vi "n4tobob1.vi"() -> ()   [LabVIEW 2014, in "Panels.lvlib"]
uses:
  Panels.lvlib
  CSlibraries-extern/DimLVEvent/DimIndicators/DimIndicators.lvlib
  CS_Core/CSSystem/CoreLib/CoreLib.lvlib
  CSlibraries/UtilityLib/UtilityLib.valueStatus.ctl
  CSlibraries/UtilityLib/UtilityLib.lvlib
  CSlibraries-extern/DimLVEvent/LVDimInterface/LVDimInterface.lvlib
  Instance           1 16Saved   n4tobob1 .vi
  CSlibraries-extern/DimLVEvent/DimIndicators/DimIndicators.numericType.ctl
  CSlibraries-extern/DimLVEvent/DimIndicators/DimIndicators.numericArrayType.ctl
  CSlibraries-extern/DimLVEvent/DimIndicators/DimIndicators.anyType.ctl
panel:
  in  "SetFileLocation_Data":T1={"data"="NOLINK", "no link"=TRUE, "quality"=-1, "timeStamp"=0.0}
  in  "LN4Accel2":bool
  in  "LN4Accel3":bool
  in  "LN4DefY":bool
  in  "LN4DefX":bool
  in  "10DegDefX":bool
  in  "ELens0":bool
  out "LN4Accel3_Mon":dbl=inf format="%.4f"
  out "LN4Accel2_Mon":dbl=inf format="%.4f"
  out "i ref out":refnum<vi>
  in  "Last Loaded File_Data":T1
  out "FileUpToDate":bool caption="Parameter Changed"
  in  "Close All Panels":bool
  in  "LN4Accel2_SetValueInfoData":T2
  in  "LN4Accel3_SetValueInfoData":T2
  in  "ELens0_SetValueInfoData":T2
  in  "LN4DefX_SetValueInfoData":T2
  in  "LN4DefY_SetValueInfoData":T2
  in  "10DegDefX_SetValueInfoData":T2
  in  "10DegDefX_SetData":T2
  in  "LN4DefY_SetData":T2
  in  "LN4DefX_SetData":T2
  in  "ELens0_SetData":T2
  in  "LN4Accel3_SetData":T2
  in  "LN4Accel2_SetData":T2
  out "Last Loaded File":string
  in  "SetFileLocation":path=path "\\\\intranet\\Files/projects/lebit/Data Exchange/data/N4tobob1Control"
  in  "10DegDefY_MonData":T3={"data"=inf, "no link"=FALSE, "quality"=1, "timeStamp"=3262371343.476}
  in  "10DegDefX_MonData":T3={"data"=inf, "no link"=FALSE, "quality"=1, "timeStamp"=3262371343.476}
  in  "LN4DefY_MonData":T3={"data"=inf, "no link"=FALSE, "quality"=1, "timeStamp"=3262371343.476}
  in  "LN4DefX_MonData":T3={"data"=inf, "no link"=FALSE, "quality"=1, "timeStamp"=3262371343.476}
  in  "ELens0_MonData":T3={"data"=inf, "no link"=FALSE, "quality"=1, "timeStamp"=3262371343.46}
  in  "LN4Accel3_MonData":T3={"data"=inf, "no link"=FALSE, "quality"=1, "timeStamp"=3262371343.46}
  in  "LN4Accel2_MonData":T3={"data"=inf, "no link"=FALSE, "quality"=1, "timeStamp"=3262371343.46}
  out "LN4DefX_Mon":dbl=inf format="%.4f"
  out "10DegDefY_Mon":dbl=inf format="%.4f"
  out "10DegDefX_Mon":dbl=inf format="%.4f"
  out "LN4DefY_Mon":dbl=inf format="%.4f"
  out "ELens0_Mon":dbl=inf format="%.4f"
  # "Parameter changed, data file is no longer up-to-date."
  # "10DegDefY"
  # "LN4Accel1 = DC8"
  # "LN4Accel4 =-5kV"
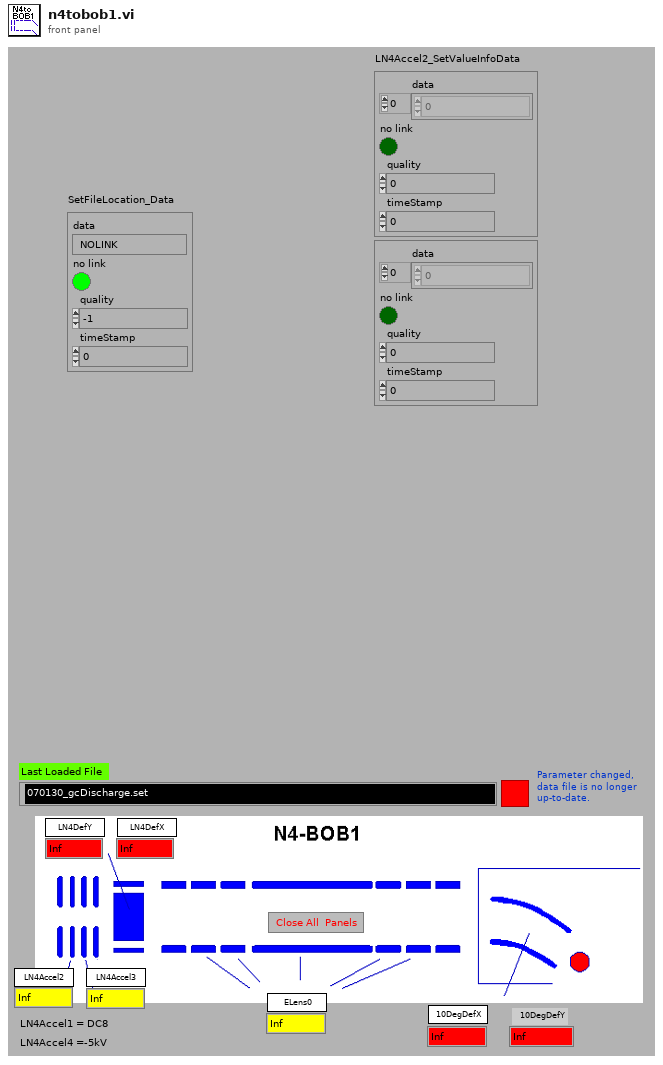
[diagram p1: front panel]
types:
  T1 = typedef "DimIndicators.lvlib/DimIndicators.anyType.ctl" = cluster{"data":string, "no link":bool, "quality":i32, "timeStamp":dbl}
  T2 = typedef "DimIndicators.lvlib/DimIndicators.numericArrayType.ctl" = cluster{"data":dbl[], "no link":bool, "quality":i32, "timeStamp":dbl}
  T3 = typedef "DimIndicators.lvlib/DimIndicators.numericType.ctl" = cluster{"data":dbl, "no link":bool, "quality":i32, "timeStamp":dbl}
  T4 = typedef "UtilityLib.lvlib/UtilityLib.valueStatus.ctl" = enum16{"no info available", "stand by/off", "on", "warning", "alarm/malfunction", "not implemented", "user action required", "important information", "system default", "control default", "indicator default", "button default"}
  T5 = cluster{"data":string, "no link":bool, "quality":i32, "timeStamp":dbl}
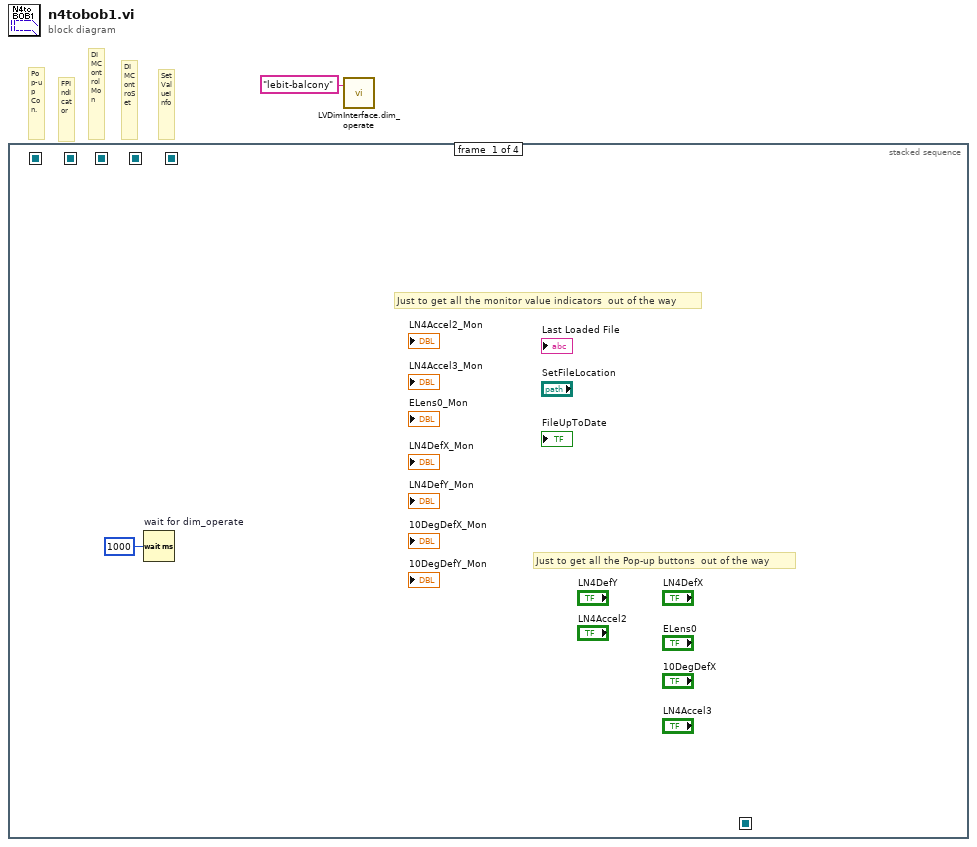
[diagram p0: block diagram]
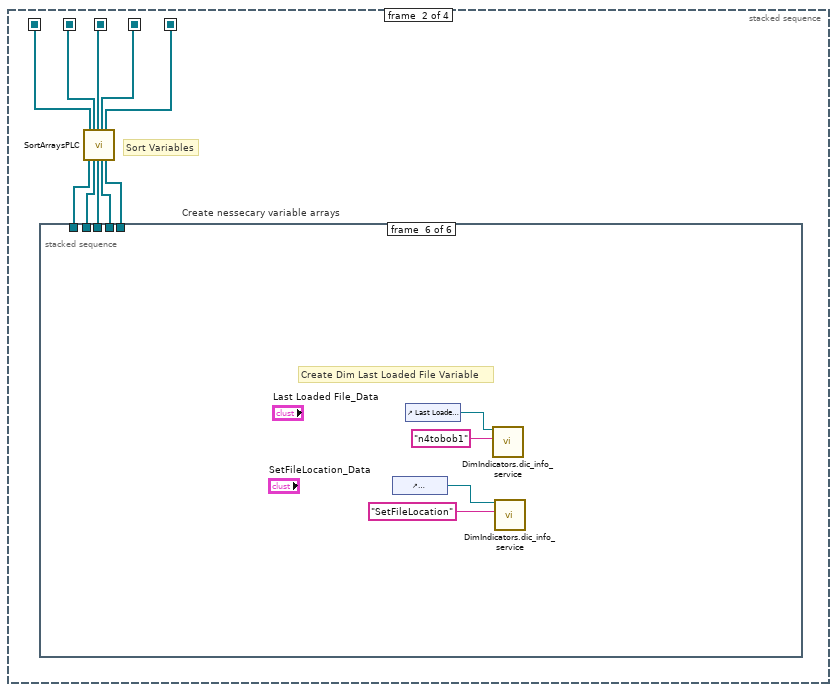
[diagram p2: hidden frame]
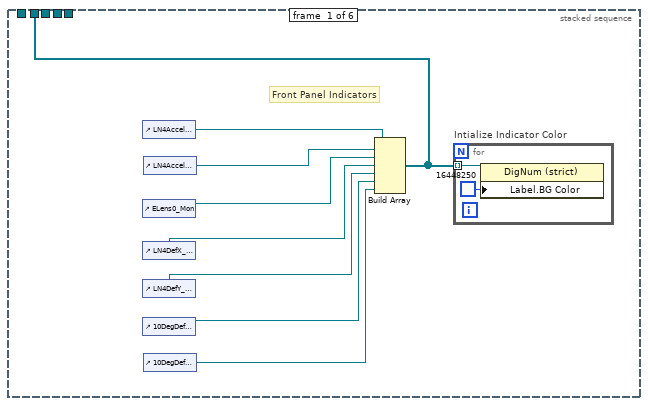
[diagram p3: hidden frame]
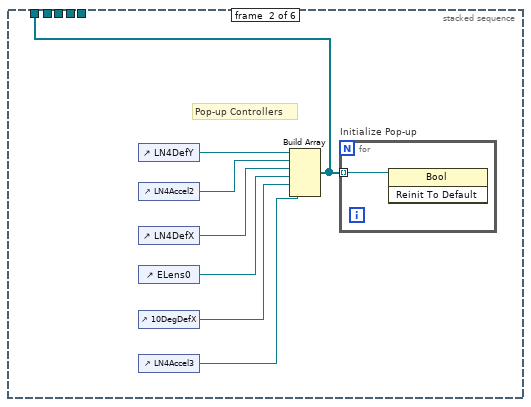
[diagram p4: hidden frame]
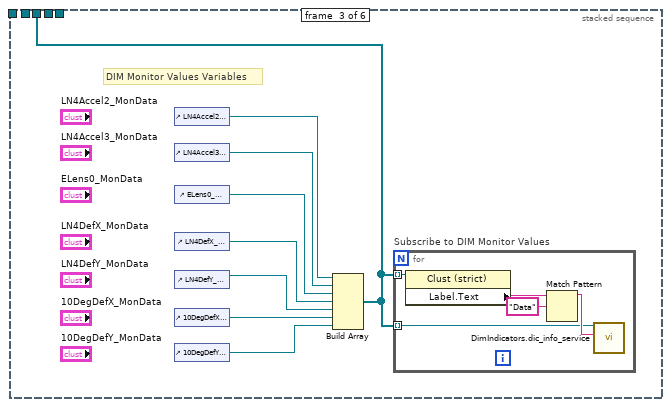
[diagram p5: hidden frame]
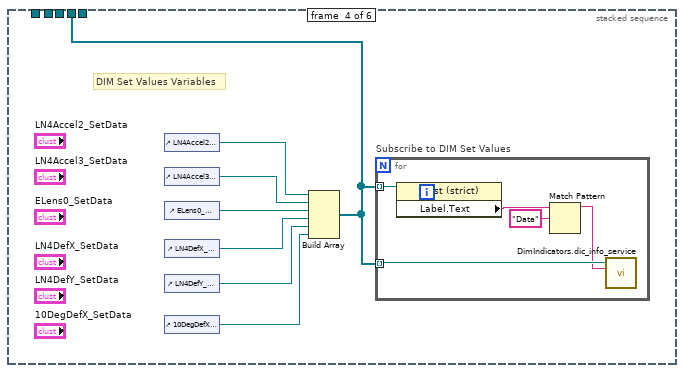
[diagram p6: hidden frame]
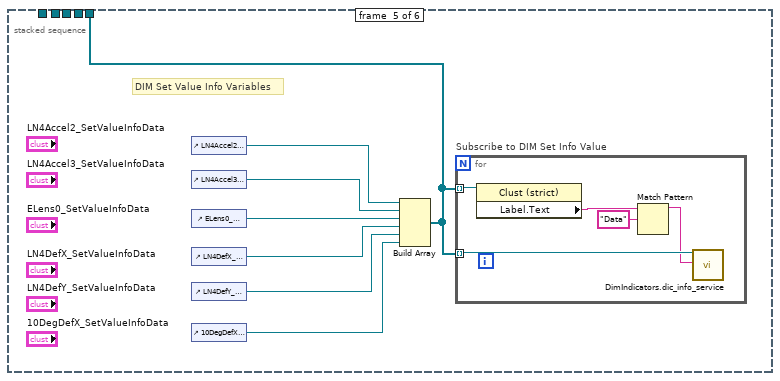
[diagram p7: hidden frame]
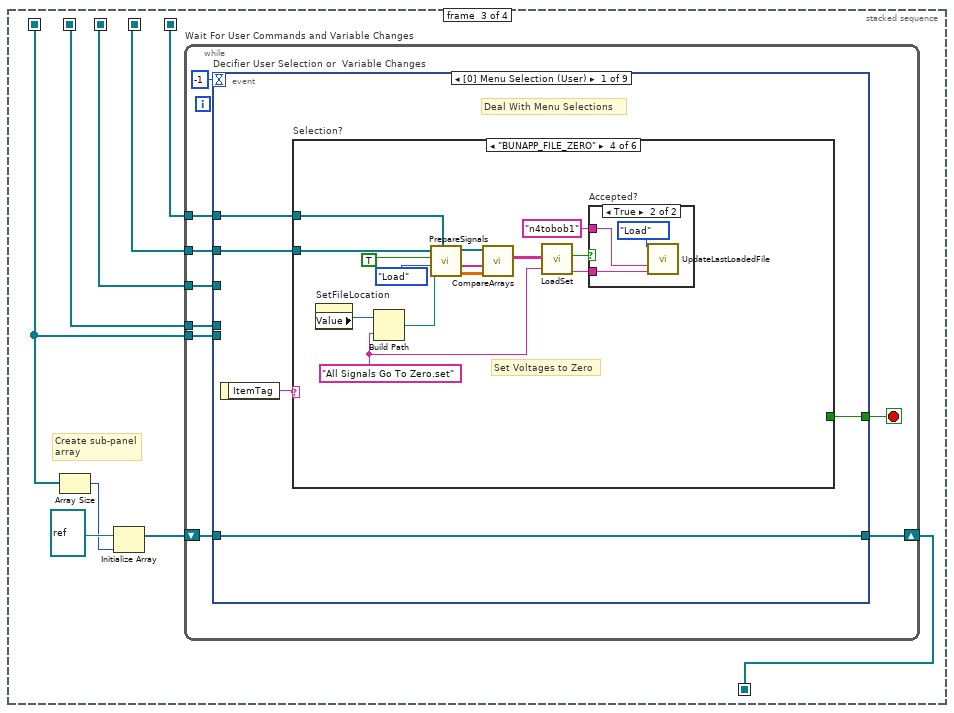
[diagram p8: hidden frame]
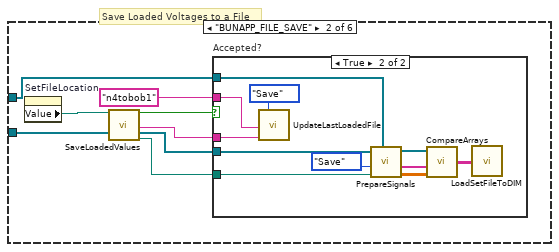
[diagram p10: hidden frame]
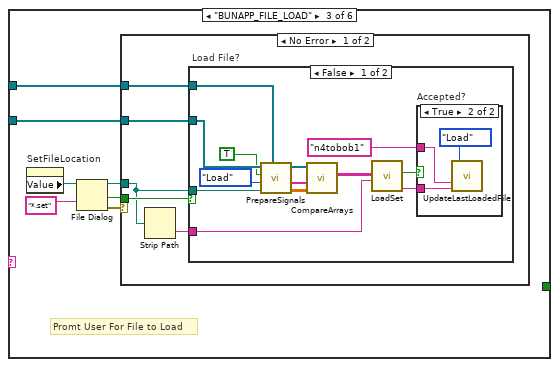
[diagram p12: hidden frame]
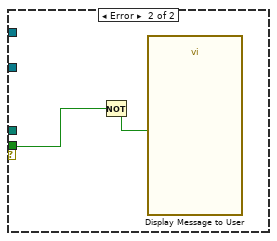
[diagram p15: hidden frame]
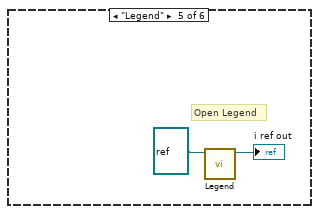
[diagram p17: hidden frame]
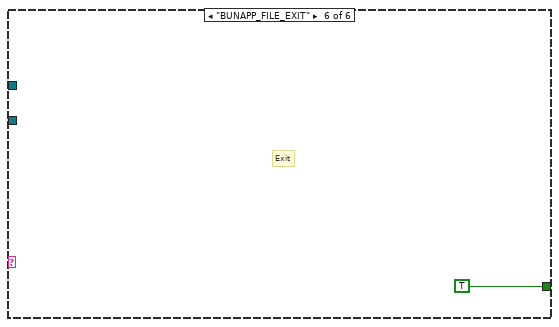
[diagram p18: hidden frame]
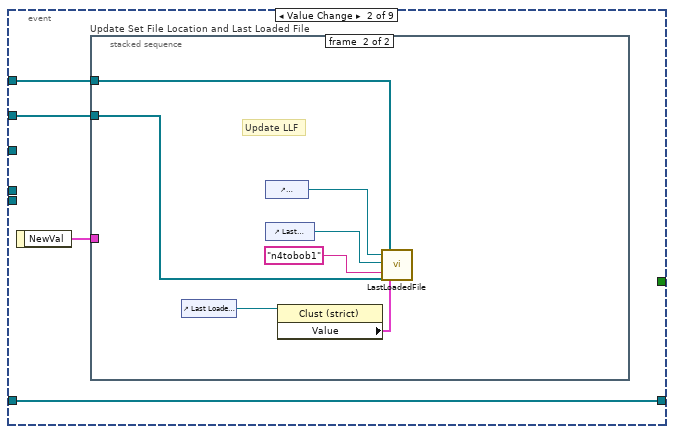
[diagram p19: hidden frame]
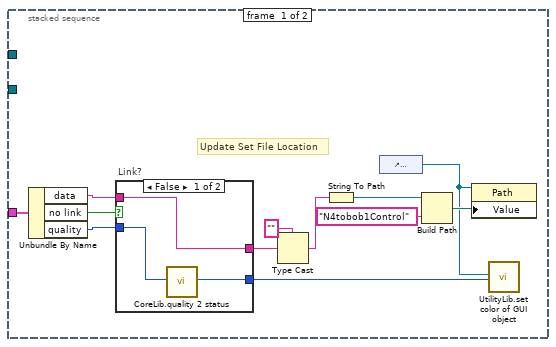
[diagram p20: hidden frame]
diagram:
  # "Pop-up Con."
  # "SetValueInfo"
  # "DIMControSet"
  # "DIMControlMon"
  # "FPIndicator"
  n1 = stacked-sequence {
    seq-local: [_ w11 _ _] -> [_ _ w77 _]
    seq-local: [_ w10 _ _] -> [_ _ w80 w273]
    seq-local: [_ _ w75 _] -> [_ _ _ w272]
    seq-local: [_ w9 _ _] -> [_ _ w74 w271]
    seq-local: [_ w8 _ _] -> [_ _ w73 w270]
    seq-local: [_ w12 _ _] -> [_ _ w72 _]
    frame #0 {
      # "Just to get all the Pop-up buttons  out of the way"
      # "Just to get all the monitor value indicators  out of the way"
      n2 = Wait (ms) "wait for dim_operate"(milliseconds to wait=u32 1000) -> ()  [unwired: 1 out]
    }
    frame #1 {
      # "Sort Variables"
      n3 = stacked-sequence "Create nessecary variable arrays" {
        tunnel: [w13 _ _ _ _ _] -> w7
        tunnel: [_ w23 _ _ _ _] -> w6
        tunnel: [_ _ w31 _ _ _] -> w5
        tunnel: [_ _ _ w44 _ _] -> w4
        tunnel: [_ _ _ _ w56 _] -> w3
        frame #0 {
          # "Front Panel Indicators"
          n4 = control-ref of="LN4Accel2_Mon"() -> (w15:refnum<vi>)
          n5 = control-ref of="ELens0_Mon"() -> (w20:refnum<vi>)
          n6 = control-ref of="LN4DefX_Mon"() -> (w19:refnum<vi>)
          n7 = control-ref of="LN4DefY_Mon"() -> (w18:refnum<vi>)
          n8 = control-ref of="10DegDefX_Mon"() -> (w17:refnum<vi>)
          n9 = control-ref of="LN4Accel3_Mon"() -> (w14:refnum<vi>)
          n10 = control-ref of="10DegDefY_Mon"() -> (w16:refnum<vi>)
          n11 = Build Array(w15, w14, w20, w19, w18, w17, w16) -> (w13:refnum<vi>[])
          n12 = for "Intialize Indicator Color" {
            tunnel: w13 -> [w22] mode=indexing
            n13 = property class="DigNum (strict)"(reference=w22, "Label.BG Color"=u32 16448250 ("Color Box")) -> ()  [unwired: 1 in, 2 out]
          }
        }
        frame #1 {
          # "Pop-up Controllers"
          n14 = control-ref of="LN4DefY"() -> (w29:refnum<vi>)
          n15 = control-ref of="LN4Accel2"() -> (w28:refnum<vi>)
          n16 = control-ref of="LN4DefX"() -> (w27:refnum<vi>)
          n17 = control-ref of="ELens0"() -> (w26:refnum<vi>)
          n18 = control-ref of="10DegDefX"() -> (w25:refnum<vi>)
          n19 = control-ref of="LN4Accel3"() -> (w24:refnum<vi>)
          n20 = Build Array(w29, w28, w27, w26, w25, w24) -> (w23:refnum<vi>[])
          n21 = for "Initialize Pop-up" {
            tunnel: w23 -> [w30] mode=indexing
            n22 = invoke class="Bool" method="Reinit To Default"(reference=w30) -> ()  [unwired: 2 in, 3 out]
          }
        }
        frame #2 {
          # "DIM Monitor Values Variables"
          n23 = control-ref of="LN4Accel2_MonData"() -> (w38:refnum<vi>)
          n24 = control-ref of="LN4Accel3_MonData"() -> (w37:refnum<vi>)
          n25 = control-ref of="ELens0_MonData"() -> (w36:refnum<vi>)
          n26 = control-ref of="LN4DefX_MonData"() -> (w35:refnum<vi>)
          n27 = control-ref of="LN4DefY_MonData"() -> (w34:refnum<vi>)
          n28 = control-ref of="10DegDefX_MonData"() -> (w33:refnum<vi>)
          n29 = control-ref of="10DegDefY_MonData"() -> (w32:refnum<vi>)
          n30 = Build Array(w38, w37, w36, w35, w34, w33, w32) -> (w31:refnum<vi>[])
          n31 = for "Subscribe to DIM Monitor Values" {
            tunnel: w31 -> [w40] mode=indexing
            tunnel: w31 -> [w39] mode=indexing
            n32 = property class="Clust (strict)"(reference=w39) -> ("Label.Text"=w42:string)  [unwired: 1 in, 2 out]
            n33 = Match Pattern(string=w42, regular expression="Data") -> (before substring=w41:string)  [unwired: 1 in, 3 out]
            n34 = call "DimIndicators.dic_info_service.vi"("controlRef"=w40, "serviceName"=w41) -> ()  [unwired: 16 in, 2 out]
          }
        }
        frame #3 {
          # "DIM Set Values Variables"
          n35 = control-ref of="LN4Accel2_SetData"() -> (w50:refnum<vi>)
          n36 = control-ref of="LN4Accel3_SetData"() -> (w49:refnum<vi>)
          n37 = control-ref of="ELens0_SetData"() -> (w48:refnum<vi>)
          n38 = control-ref of="LN4DefX_SetData"() -> (w47:refnum<vi>)
          n39 = control-ref of="LN4DefY_SetData"() -> (w46:refnum<vi>)
          n40 = control-ref of="10DegDefX_SetData"() -> (w45:refnum<vi>)
          n41 = Build Array(w50, w49, w48, w47, w46, w45) -> (w44:refnum<vi>[])
          n42 = for "Subscribe to DIM Set Values" {
            tunnel: w44 -> [w51] mode=indexing
            tunnel: w44 -> [w55] mode=indexing
            n43 = property class="Clust (strict)"(reference=w51) -> ("Label.Text"=w54:string)  [unwired: 1 in, 2 out]
            n44 = Match Pattern(string=w54, regular expression="Data") -> (before substring=w52:string)  [unwired: 1 in, 3 out]
            n45 = call "DimIndicators.dic_info_service.vi"("controlRef"=w55, "serviceName"=w52) -> ()  [unwired: 16 in, 2 out]
          }
        }
        frame #4 {
          # "DIM Set Value Info Variables"
          n46 = control-ref of="LN4Accel2_SetValueInfoData"() -> (w62:refnum<vi>)
          n47 = control-ref of="LN4Accel3_SetValueInfoData"() -> (w61:refnum<vi>)
          n48 = control-ref of="ELens0_SetValueInfoData"() -> (w60:refnum<vi>)
          n49 = control-ref of="LN4DefX_SetValueInfoData"() -> (w59:refnum<vi>)
          n50 = control-ref of="LN4DefY_SetValueInfoData"() -> (w58:refnum<vi>)
          n51 = control-ref of="10DegDefX_SetValueInfoData"() -> (w57:refnum<vi>)
          n52 = Build Array(w62, w61, w60, w59, w58, w57) -> (w56:refnum<vi>[])
          n53 = for "Subscribe to DIM Set Info Value" {
            tunnel: w56 -> [w63] mode=indexing
            tunnel: w56 -> [w67] mode=indexing
            n54 = property class="Clust (strict)"(reference=w63) -> ("Label.Text"=w66:string)  [unwired: 1 in, 2 out]
            n55 = Match Pattern(string=w66, regular expression="Data") -> (before substring=w64:string)  [unwired: 1 in, 3 out]
            n56 = call "DimIndicators.dic_info_service.vi"("controlRef"=w67, "serviceName"=w64) -> ()  [unwired: 16 in, 2 out]
          }
        }
        frame #5 {
          # "Create Dim Last Loaded File Variable"
          n57 = control-ref of="SetFileLocation_Data"() -> (w71:refnum<vi>)
          n58 = control-ref of="Last Loaded File_Data"() -> (w69:refnum<vi>)
          n59 = call "DimIndicators.dic_info_service.vi"("controlRef"=w69, "serviceName"="n4tobob1" ("string")) -> ()  [unwired: 16 in, 2 out]
          n60 = call "DimIndicators.dic_info_service.vi"("controlRef"=w71, "serviceName"="SetFileLocation" ("string")) -> ()  [unwired: 16 in, 2 out]
        }
      }
      n61 = call "SortArraysPLC.vi"("Pop-up Con."=w6, "FPIndicator in"=w7, "DIMControlMon"=w5, "DIMControSet"=w4, "SetValueInfo"=w3) -> ("Pop-up Con. out"=w12:refnum<vi>[], "FPIndicator out"=w11:refnum<vi>[], "DIMControlMon out"=w10:refnum<vi>[], "DIMControSet out"=w9:refnum<vi>[], "SetValueInfo out"=w8:refnum<vi>[])  [unwired: 18 in]
    }
    frame #2 {
      # "Create sub-panel\narray"
      n62 = Array Size(array=w72) -> (size(s)=w76:i32)
      n63 = Initialize Array(refnum<vi> refnum ("vi reference"), w76) -> (w79:refnum<vi>[])
      n64 = while "Wait For User Commands and Variable Changes" {
        tunnel: w80 -> [w88]
        tunnel: w77 -> [w87]
        shift-right: [w85] -> w75
        shift-left: w79 -> [w86]
        tunnel: w74 -> [w84]
        tunnel: w73 -> [w83]
        tunnel: w72 -> [w81]
        stop <- w89 stop-if-true
        n65 = event "Decifier User Selection or  Variable Changes" shown="[0] Menu Selection (User)" {
          selector: _ -> [_ _ _ _ _ _ _ _ _]
          dyn-events: _ -> [_ _ _ _ _ _ _ _ _]
          timeout: -1 -> [_ _ _ _ _ _ _ _ _]
          tunnel: [w91 _ _ _ _ _ _ _ TRUE ("stop")] -> w89
          tunnel: w88 -> [_ _ _ w203 _ _ _ _ w246]
          tunnel: w87 -> [_ _ _ w202 _ _ _ _ _]
          tunnel: w86 -> [w94 w165 w198 w205 w223 w231 w238 w244 w245]
          tunnel: [w94 w165 w198 w205 w223 w229 w236 w244 _] -> w85
          tunnel: w84 -> [w92 w166 w195 _ w221 _ _ _ w247]
          tunnel: w83 -> [w90 w164 w192 _ _ _ _ _ w248]
          tunnel: w81 -> [_ _ _ _ _ w225 _ _ _]
          event Menu Selection (User) {
            # "Deal With Menu Selections"
            n66 = event-data() -> ("ItemTag"=w93:string)  [unwired: 1 in]
            n67 = case "Selection?" shown="\"BUNAPP_FILE_ZERO\"" w93 {
              tunnel: w92 -> [_ w99 w119 w157 _ _]
              tunnel: [_ _ _ _ _ TRUE ("stop")] -> w91
              tunnel: w90 -> [_ w95 w114 w144 _ _]
              frame "False", Default {
              }
              frame "BUNAPP_FILE_SAVE" {
                # "Save Loaded Voltages to a File"
                n68 = property on="SetFileLocation" class="Path"() -> ("Value"=w100:path)  [unwired: 2 in, 2 out]
                n69 = call "SaveLoadedValues.vi"("Panel Location?"=w100, "DIMControlSet in"=w99) -> ("File Saved?"=w101:bool, "File Name"=w98:string, "DIMControlSet out"=w96:refnum<vi>[], "Path"=w97:path)  [unwired: 14 in]
                n70 = case "Accepted?" shown="True" w101 {
                  tunnel: w98 -> [_ w111]
                  tunnel: "n4tobob1" ("string") -> [_ w113]
                  tunnel: w96 -> [_ w112]
                  tunnel: w97 -> [_ w110]
                  tunnel: w95 -> [_ w104]
                  frame False {
                  }
                  frame True {
                    n71 = call "UpdateLastLoadedFile.vi"("LoadOrSave"=enum16{"Load", "Save"}."Save", "GUIName"=w113, "FileNameIn"=w111) -> ()  [unwired: 13 in]
                    n72 = call "PrepareSignals.vi"("SetValueInfo in"=w104, "setfile path"=w110, "Enum"=enum16{"Save", "Load"}."Save", "DIMControSet in"=w112) -> ("indexed loaded Array"=w108:dbl[][], "Name Array"=w109:string[], "DIMControSet out"=w107:refnum<vi>[])  [unwired: 5 in]
                    n73 = call "CompareArrays.vi"("indexed loaded Array"=w108, "Name Array"=w109, "DIMControSet"=w107) -> ("Table for loading values"=w106:string[][])  [unwired: 4 in]
                    n74 = call "LoadSetFileToDIM.vi"("output array"=w106) -> ()  [unwired: 2 in]
                  }
                }
              }
              frame "BUNAPP_FILE_LOAD" {
                # "Promt User For File to Load"
                n75 = property on="SetFileLocation" class="Path"() -> ("Value"=w116:path)  [unwired: 2 in, 2 out]
                n76 = File Dialog(6:"*.set" ("pattern (all files)"), 11:w116) -> (0:w115:errorcluster, 1:w120:bool, 3:w117:path)  [unwired: 5 in, 1 out]
                n77 = case shown="No Error" w115 {
                  tunnel: w120 -> [w125 w142]
                  tunnel: w119 -> [w124 _]
                  tunnel: w117 -> [w122 _]
                  tunnel: w114 -> [w121 _]
                  frame No Error {
                    n78 = Strip Path(path=w122) -> (name=w123:string)  [unwired: 1 out]
                    n79 = case "Load File?" shown="False" w125 {
                      tunnel: w124 -> [w138 _]
                      tunnel: w123 -> [w132 _]
                      tunnel: w122 -> [w133 _]
                      tunnel: w121 -> [w126 _]
                      frame False {
                        n80 = call "PrepareSignals.vi"("SetValueInfo in"=w126, "setfile path"=w133, "Enum"=enum16{"Save", "Load"}."Load", "Display Message to \nUser"=TRUE ("Display Message to \nUser"), "DIMControSet in"=w138) -> ("indexed loaded Array"=w136:dbl[][], "Name Array"=w135:string[], "DIMControSet out"=w137:refnum<vi>[])  [unwired: 4 in]
                        n81 = call "CompareArrays.vi"("indexed loaded Array"=w136, "Name Array"=w135, "DIMControSet"=w137) -> ("Table for loading values"=w134:string[][])  [unwired: 4 in]
                        n82 = call "LoadSet.vi"("File Name In"=w132, "output array"=w134) -> ("File Name out"=w131:string, "Accepted"=w130:bool)  [unwired: 8 in]
                        n83 = case "Accepted?" shown="True" w130 {
                          tunnel: w131 -> [_ w141]
                          tunnel: "n4tobob1" ("string") -> [_ w140]
                          frame False {
                          }
                          frame True {
                            n84 = call "UpdateLastLoadedFile.vi"("LoadOrSave"=enum16{"Load", "Save"}."Load", "GUIName"=w140, "FileNameIn"=w141) -> ()  [unwired: 13 in]
                          }
                        }
                      }
                      frame True {
                      }
                    }
                  }
                  frame Error {
                    n85 = Not(x=w142) -> (.not. x?=w143:bool)
                    n86 = call "Display Message to User"("Enable"=w143) -> ()  [unwired: 9 in, 2 out]
                  }
                }
              }
              frame "BUNAPP_FILE_ZERO" {
                w148 = "All Signals Go To Zero.set" ("File Name")
                # "Set Voltages to Zero"
                n87 = property on="SetFileLocation" class="Path"() -> ("Value"=w146:path)  [unwired: 2 in, 2 out]
                n88 = Build Path(base path=w146, name or relative path=w148) -> (appended path=w147:path)
                n89 = call "PrepareSignals.vi"("SetValueInfo in"=w144, "setfile path"=w147, "Enum"=enum16{"Save", "Load"}."Load", "Display Message to \nUser"=TRUE ("Display Message to \nUser"), "DIMControSet in"=w157) -> ("indexed loaded Array"=w155:dbl[][], "Name Array"=w154:string[], "DIMControSet out"=w156:refnum<vi>[])  [unwired: 4 in]
                n90 = call "CompareArrays.vi"("indexed loaded Array"=w155, "Name Array"=w154, "DIMControSet"=w156) -> ("Table for loading values"=w153:string[][])  [unwired: 4 in]
                n91 = call "LoadSet.vi"("File Name In"=w148, "output array"=w153) -> ("File Name out"=w151:string, "Accepted"=w152:bool)  [unwired: 8 in]
                n92 = case "Accepted?" shown="True" w152 {
                  tunnel: w151 -> [_ w160]
                  tunnel: "n4tobob1" ("string") -> [_ w159]
                  frame False {
                  }
                  frame True {
                    n93 = call "UpdateLastLoadedFile.vi"("LoadOrSave"=enum16{"Load", "Save"}."Load", "GUIName"=w159, "FileNameIn"=w160) -> ()  [unwired: 13 in]
                  }
                }
              }
              frame "Legend" {
                # "Open Legend"
                n94 = call "Legend.vi"("i ref in"=refnum<vi> refnum) -> ("i ref out"=→"i ref out":refnum<vi>)  [unwired: 10 in]
              }
              frame "BUNAPP_FILE_EXIT" {
                # "Exit"
              }
            }
          }
          event Value Change {
            n95 = event-data() -> ("NewVal"=w167:T1)  [unwired: 1 in]
            n96 = stacked-sequence "Update Set File Location and Last Loaded File" {
              tunnel: w167 -> [w169 _]
              tunnel: w166 -> [_ w189]
              tunnel: w164 -> [_ w185]
              frame #0 {
                # "Update Set File Location"
                n97 = Unbundle By Name(w169) -> ("data"=w178:string, "no link"=w177:bool, "quality"=w176:i32)
                n98 = case "Link?" shown="False" w177 {
                  tunnel: w176 -> [w182 _]
                  tunnel: [w181 UtilityLib.valueStatus."no info available" ("valueStatus")] -> w179
                  tunnel: w178 -> [w180 _]
                  tunnel: [w180 w183] -> w174
                  frame False {
                    n99 = call "CoreLib.quality 2 status.vi"("quality"=w182) -> ("valueStatus"=w181:T4)  [unwired: 18 in]
                  }
                  frame True {
                    n100 = call "EmptyString.vi"() -> ("String"=w183:string)
                  }
                }
                n101 = Type Cast(type="" ("regular expression"), x=w174) -> (*(type *) &x=w173:string)
                n102 = String To Path(string=w173) -> (path=w170:path)
                n103 = control-ref of="SetFileLocation"() -> (w168:refnum<vi>)
                n104 = Build Path(base path=w170, name or relative path="N4tobob1Control") -> (appended path=w171:path)
                n105 = property class="Path"(reference=w168, "Value"=w171) -> ()  [unwired: 1 in, 2 out]
                n106 = call "UtilityLib.set color of GUI object.vi"("GUI object Ref"=w168, "valueStatus"=w179) -> ()  [unwired: 17 in, 1 out]
              }
              frame #1 {
                # "Update LLF"
                n107 = control-ref of="Last Loaded File_Data"() -> (w190:refnum<vi>)
                n108 = control-ref of="SetFileLocation"() -> (w187:refnum<vi>)
                n109 = control-ref of="Last Loaded File"() -> (w188:refnum<vi>)
                n110 = property class="Clust (strict)"(reference=w190) -> ("Value"=w191:T5)  [unwired: 1 in, 2 out]
                n111 = call "LastLoadedFile.vi"("SetFileLocation"=w187, "Last Loaded File"=w188, "GUIName"="n4tobob1", "DIMControSet in"=w189, "SetValueInfo in"=w185, "NewVal"=w191) -> ()  [unwired: 14 in]
              }
            }
          }
          event Value Change {
            # "Update Last Loaded File"
            n112 = event-data() -> ("NewVal"=w196:T1)  [unwired: 1 in]
            n113 = control-ref of="Last Loaded File"() -> (w193:refnum<vi>)
            n114 = control-ref of="SetFileLocation"() -> (w194:refnum<vi>)
            n115 = call "LastLoadedFile.vi"("SetFileLocation"=w194, "Last Loaded File"=w193, "GUIName"="n4tobob1", "DIMControSet in"=w195, "SetValueInfo in"=w192, "NewVal"=w196) -> ()  [unwired: 14 in]
          }
          event Value Change {
            # "Find Monitor Value Index"
            # "Updating a Monitor Value"
            n116 = event-data() -> ("CtlRef"=w201:refnum<vi>, "NewVal"=w206:T3)  [unwired: 1 in, 4 out]
            n117 = Search 1D Array(1D array=w203, element=w201) -> (index of element=w204:i32)  [unwired: 1 in]
            n118 = Index Array(array=w202, index=w204) -> (element=w200:refnum<vi>)
            n119 = Not A Number/Path/Refnum?(number/path/refnum=w200) -> (NaN/Path/Refnum?=w199:bool)
            n120 = case "Indicator does not exists?" shown="False" w199 {
              tunnel: w206 -> [_ w213]
              tunnel: w200 -> [_ w207]
              frame True {
              }
              frame False {
                n121 = Unbundle By Name(w213) -> ("data"=w209:dbl, "no link"=w210:bool, "quality"=w212:i32)
                n122 = case shown="True" w210 {
                  tunnel: w212 -> [w216 _]
                  tunnel: [w215 UtilityLib.valueStatus."no info available" ("valueStatus")] -> w211
                  tunnel: w209 -> [w214 _]
                  tunnel: [w214 inf] -> w208
                  frame False {
                    n123 = call "CoreLib.quality 2 status.vi"("quality"=w216) -> ("valueStatus"=w215:T4)  [unwired: 18 in]
                  }
                  frame True {
                  }
                }
                n124 = property class="DigNum (strict)"(reference=w207, "Value"=w208) -> ()  [unwired: 1 in, 2 out]
                n125 = call "TextColor.vi"("valueStatus"=w211, "reference"=w207) -> ()  [unwired: 10 in]
              }
            }
          }
          event Value Change {
            n126 = event-data() -> ("CtlRef"=w220:refnum<vi>)  [unwired: 1 in, 5 out]
            n127 = property on="FileUpToDate" class="Bool (strict)"() -> ("Value"=w219:bool)  [unwired: 2 in, 2 out]
            n128 = call "FileUpToDate.vi"("FileUpToDate in"=w219, "DIMControSet out"=w221, "CtlRef"=w220) -> ("FileUpToDate out"=w222:bool)  [unwired: 16 in]
            n129 = property on="FileUpToDate" class="Bool (strict)"("Value"=w222) -> ()  [unwired: 2 in, 2 out]
          }
          event "ELens0", "10DegDefX", "LN4DefX", "LN4DefY", "LN4Accel3", "LN4Accel2": Value Change {
            # "Find sub-panel index"
            # "opening or closing a sub-panel"
            n130 = event-data() -> ("CtlRef"=w224:refnum<vi>)  [unwired: 1 in, 3 out]
            n131 = Search 1D Array(1D array=w225, element=w224) -> (index of element=w230:i32)  [unwired: 1 in]
            n132 = Index Array(array=w231, index=w230) -> (element=w228:refnum<vi>)
            n133 = invoke class="Bool" method="Reinit To Default"(reference=w224) -> ()  [unwired: 2 in, 3 out]
            n134 = property class="VI"(reference=w228) -> ("Front Panel.Open"=w227:bool)  [unwired: 1 in, 2 out]
            n135 = case "Panel Already Open?" shown="False" w227 {
              tunnel: w224 -> [w232 _]
              tunnel: w228 -> [_ w235]
              tunnel: [w233 refnum<vi> refnum ("vi reference")] -> w226
              frame False {
                n136 = call "OpenPanel.vi"("CtlRef"=w232) -> ("vi reference"=w233:refnum<vi>)  [unwired: 2 in]
              }
              frame True {
                n137 = call "PanelClose.vi"("vi reference"=w235) -> ()
              }
            }
            n138 = Replace Array Subset(array=w231, new element=w226, index=w230) -> (w229:refnum<vi>[])
          }
          event "Close All Panels": Value Change {
            n139 = event-data() -> ()  [unwired: 1 in, 6 out]
            n140 = case "Close Open Panels?" shown="True" "Close All Panels" {
              tunnel: w238 -> [w239 w241]
              tunnel: [w239 w240] -> w236
              frame False {
              }
              frame True {
                n141 = for "Close Open Panels" {
                  tunnel: w241 -> [w243] mode=indexing
                  tunnel: w241 -> [w242]
                  tunnel: [w242] -> w240
                  n142 = call "PanelClose.vi"("vi reference"=w243) -> ()
                }
              }
            }
          }
          event Timeout {
            # "Timeout"
            n143 = event-data() -> ()  [unwired: 1 in, 3 out]
          }
          event Panel Close? {
            n144 = event-data() -> ()  [unwired: 1 in, 4 out]
            n145 = stacked-sequence {
              tunnel: w248 -> [w253 _]
              tunnel: w247 -> [w252 _]
              tunnel: w246 -> [w251 _]
              tunnel: w245 -> [w255 _]
              frame #0 {
                # "Release DIM Services"
                n146 = for "Close Open Panels" {
                  tunnel: w255 -> [w265] mode=indexing
                  n147 = call "PanelClose.vi"("vi reference"=w265) -> ()
                }
                n148 = for "For Each Service" {
                  tunnel: w252 -> [w260] mode=indexing
                  n149 = Not A Number/Path/Refnum?(number/path/refnum=w260) -> (NaN/Path/Refnum?=w259:bool)
                  n150 = case "Not a Reference?" shown="False" w259 {
                    tunnel: w260 -> [w261 _]
                    frame False {
                      n151 = call "DimIndicators.dic_release_service.vi"("controlRef"=w261) -> ()  [unwired: 18 in, 1 out]
                    }
                    frame True {
                    }
                  }
                }
                n152 = for "For Each Service" {
                  tunnel: w251 -> [w257] mode=indexing
                  n153 = Not A Number/Path/Refnum?(number/path/refnum=w257) -> (NaN/Path/Refnum?=w256:bool)
                  n154 = case "Not a Reference?" shown="False" w256 {
                    tunnel: w257 -> [w258 _]
                    frame False {
                      n155 = call "DimIndicators.dic_release_service.vi"("controlRef"=w258) -> ()  [unwired: 18 in, 1 out]
                    }
                    frame True {
                    }
                  }
                }
                n156 = for "For Each Service" {
                  tunnel: w253 -> [w263] mode=indexing
                  n157 = Not A Number/Path/Refnum?(number/path/refnum=w263) -> (NaN/Path/Refnum?=w262:bool)
                  n158 = case "Not a Reference?" shown="False" w262 {
                    tunnel: w263 -> [w264 _]
                    frame False {
                      n159 = call "DimIndicators.dic_release_service.vi"("controlRef"=w264) -> ()  [unwired: 18 in, 1 out]
                    }
                    frame True {
                    }
                  }
                }
                n160 = control-ref of="SetFileLocation_Data"() -> (w250:refnum<vi>)
                n161 = control-ref of="Last Loaded File_Data"() -> (w254:refnum<vi>)
                n162 = call "DimIndicators.dic_release_service.vi"("controlRef"=w254) -> ()  [unwired: 18 in, 1 out]
                n163 = call "DimIndicators.dic_release_service.vi"("controlRef"=w250) -> ()  [unwired: 18 in, 1 out]
              }
              frame #1 {
                # "Close Front Panel"
                n164 = Current VI's Path() -> (path=w266:path)
                n165 = Open VI Reference(vi path=w266) -> (vi reference=w268:refnum<vi>, error out=w269:errorcluster)  [unwired: 5 in]
                n166 = property class="VI"(reference=w268, error in=w269, "Front Panel Window:Open"=FALSE) -> ()  [unwired: 2 out]
              }
            }
            n167 = event-data() -> ()  [unwired: 2 in, 1 out]
          }
        }
      }
    }
    frame #3 {
      n168 = stacked-sequence {
        tunnel: w273 -> [w275 _ _]
        tunnel: w272 -> [w279 _ _]
        tunnel: w271 -> [w276 _ _]
        tunnel: w270 -> [w277 _ _]
        frame #0 {
          # "Release DIM Services"
          n169 = control-ref of="SetFileLocation_Data"() -> (w274:refnum<vi>)
          n170 = control-ref of="Last Loaded File_Data"() -> (w278:refnum<vi>)
          n171 = call "DimIndicators.dic_release_service.vi"("controlRef"=w274) -> ()  [unwired: 18 in, 1 out]
          n172 = call "DimIndicators.dic_release_service.vi"("controlRef"=w278) -> ()  [unwired: 18 in, 1 out]
          n173 = for "For Each Service" {
            tunnel: w277 -> [w287] mode=indexing
            n174 = Not A Number/Path/Refnum?(number/path/refnum=w287) -> (NaN/Path/Refnum?=w286:bool)
            n175 = case "Not a Reference?" shown="False" w286 {
              tunnel: w287 -> [w288 _]
              frame False {
                n176 = call "DimIndicators.dic_release_service.vi"("controlRef"=w288) -> ()  [unwired: 18 in, 1 out]
              }
              frame True {
              }
            }
          }
          n177 = for "For Each Service" {
            tunnel: w276 -> [w284] mode=indexing
            n178 = Not A Number/Path/Refnum?(number/path/refnum=w284) -> (NaN/Path/Refnum?=w283:bool)
            n179 = case "Not a Reference?" shown="False" w283 {
              tunnel: w284 -> [w285 _]
              frame False {
                n180 = call "DimIndicators.dic_release_service.vi"("controlRef"=w285) -> ()  [unwired: 18 in, 1 out]
              }
              frame True {
              }
            }
          }
          n181 = for "For Each Service" {
            tunnel: w275 -> [w281] mode=indexing
            n182 = Not A Number/Path/Refnum?(number/path/refnum=w281) -> (NaN/Path/Refnum?=w280:bool)
            n183 = case "Not a Reference?" shown="False" w280 {
              tunnel: w281 -> [w282 _]
              frame False {
                n184 = call "DimIndicators.dic_release_service.vi"("controlRef"=w282) -> ()  [unwired: 18 in, 1 out]
              }
              frame True {
              }
            }
          }
          n185 = for "Close Open Panels" {
            tunnel: w279 -> [w289] mode=indexing
            n186 = call "PanelClose.vi"("vi reference"=w289) -> ()
          }
        }
        frame #1 {
          # "Close Front Panel"
          n187 = Current VI's Path() -> (path=w293:path)
          n188 = Open VI Reference(vi path=w293) -> (vi reference=w291:refnum<vi>, error out=w290:errorcluster)  [unwired: 5 in]
          n189 = property class="VI"(reference=w291, error in=w290, "Front Panel Window:Open"=FALSE) -> ()  [unwired: 2 out]
        }
        frame #2 {
          # "Stop Panel"
          n190 = Stop(stop? (T)=TRUE) -> ()
        }
      }
    }
  }
  n191 = call "LVDimInterface.dim_operate.vi"("DNSNode"="lebit-balcony" ("DNS node")) -> ()  [unwired: 19 in]
